vi "Tektronix DPO MSO 2000 4000 Series Create Arbitrary Waveform Example.vi"() -> ()   [LabVIEW 2016]
doc: "This example illustrates how to configure and output an arbitrary waveform.\n\n<B>Notes:</B>\n(1) This VI is available for MDO3000 Series only.\n\n(2) Requires the MDO3AFG option to be installed."
uses:
  <instrlib>/Tektronix DPO MSO 2000 4000 Series/Tektronix DPO MSO 2000 4000 Series.lvlib
panel:
  in  "VISA Resource Name":refnum<visa-resource-name>
  in  "Frequency (100000 Hz)":dbl=100000.0
  in  "Amplitude (0.5 V)":dbl=0.5
  in  "Waveform Data":dbl[](array[numeric])=[0.1, 0.2, 0.5, 0.1, -0.2]
  in  "Impedance (1: High Impedance)":i32(ring)=1 items=["50 Ohms", "High Impedance"]
  # "(C) 2006 - 2016. National Instruments Corporation. ALL RIGHTS RESERVED."
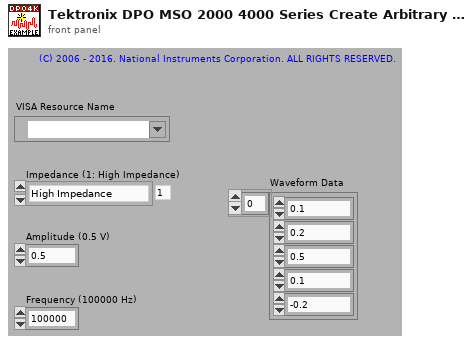
[diagram p1: front panel]
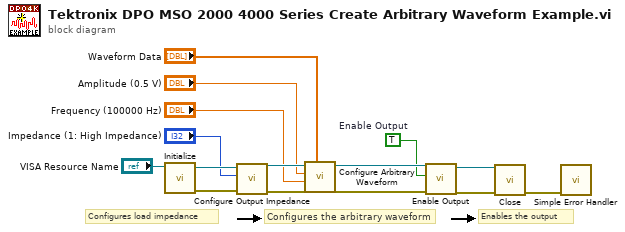
[diagram p0: block diagram]
diagram:
  w4 = TRUE  # Enable Output
  # "Enables the output"
  # "Configures the arbitrary waveform"
  # "Configures load impedance"
  n1 = call <instrlib>:"Initialize.vi"("VISA resource name"="VISA Resource Name") -> ("error out"=w13:errorcluster, "VISA resource name out"=w14:refnum<visa-resource-name>)  [unwired: 9 in]
  n2 = call <instrlib>:"Configure Output Impedance.vi"("error in (no error)"=w13, "Impedance (1: High Impedance)"="Impedance (1: High Impedance)", "VISA resource name"=w14) -> ("error out"=w11:errorcluster, "VISA resource name out"=w12:refnum<visa-resource-name>)  [unwired: 7 in]
  n3 = call <instrlib>:"Configure Arbitrary Waveform.vi"("Waveform Data"="Waveform Data", "error in (no error)"=w11, "Frequency (100000 Hz)"="Frequency (100000 Hz)", "Amplitude (0.5 V)"="Amplitude (0.5 V)", "VISA resource name"=w12) -> ("error out"=w9:errorcluster, "VISA resource name out"=w10:refnum<visa-resource-name>)  [unwired: 5 in]
  n4 = call <instrlib>:"Enable Output.vi"("error in (no error)"=w9, "Enable Output (F: Disable)"=w4, "VISA resource name"=w10) -> ("error out"=w7:errorcluster, "VISA resource name out"=w8:refnum<visa-resource-name>)  [unwired: 7 in]
  n5 = call <instrlib>:"Close.vi"("error in (no error)"=w7, "VISA resource name"=w8) -> ("error out"=w15:errorcluster)  [unwired: 9 in]
  n6 = call <vilib>:"Simple Error Handler.vi"("error in (no error)"=w15) -> ()  [unwired: 4 in, 5 out]
